vi "detect_noise.vi"(9 "threshold":dbl, 10 "i1-i3":dbl, 11 "i4-i2":dbl) -> (3 "is signal":bool)   [LabVIEW 2011]
doc: "Compares the sum of the absolute values of i4-i2 and i1-3. For reflections in the mirror that show a phase shifted fringe pattern, this sum is large while for static signals (background, mounts, etc.) this value only fluctuates a little bit. The phase for those pixels is set to zero. \nWithout this step, the divsion of i4-i2/i1-3 gives completely random values that can be extremely large and create noise in the phase map that will disturb the phase unwrapping."
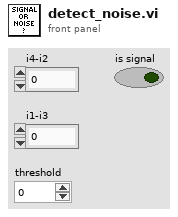
[diagram p1: front panel]
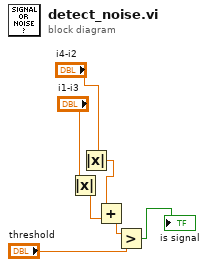
[diagram p0: block diagram]
diagram:
  n1 = Absolute Value(x="i1-i3") -> (abs(x)=w4:dbl)
  n2 = Absolute Value(x="i4-i2") -> (abs(x)=w3:dbl)
  n3 = Add(x=w3, y=w4) -> (x+y=w5:dbl)
  n4 = Greater?(x=w5, y="threshold") -> (0:→"is signal":bool)
